vi "UHR-Fleezers Control (host) - 12.0_test_fpga_connection.vi"() -> ()   [LabVIEW 2014] (continued)
  out "Left Y":i8(slide) scale=-128.0..127.0
  out "Left X":i8(slide) scale=-128.0..127.0
  out "Right Y":i8(slide) scale=-128.0..127.0
  out "Right X":i8(slide) scale=-128.0..127.0
  out "X":bool
  out "Y":bool
  out "A":bool
  out "B":bool
  out "RB":bool
  out "LB":bool
  out "R":bool
  out "L":bool
  out "D":bool
  out "U":bool
  out "Left stick button":bool
  out "FAST Z":bool
  out "FAST X-Y":bool
  in  "XY Wait time":string="125"
  in  "Z Wait time":string="120"
  # "After"
  # "During"
  # "Trap On?"
  # "BD Flow ON?"
  # "Samp Flow ON?"
  # "Fish after\nbreak?"
  # "Thresholds (nm)"
  # "From FX (nm)"
  # "Break?"
  # "Multiple"
  # "Bad fit"
  # "Hysteresis"
  # "Trap Trig. Fl.?"
  # "1"
  # "2"
  # "Fl. Down"
  # "Fl. Up"
  # "Bead sep"
  # "Trap Display:"
  # "APD Display:"
  # "Trap Manipulation"
  # "Data Saving"
  # "DAQ"
  # "Bead Calibration"
  # "Tether screen"
  # "Bottom Pump (#1)"
  # "Central Sample Channels"
  # "Top Pump (#3)"
  # "Rate param is ul/h\nVolume param is ul"
  # "Chemyx Pump 2"
  # "Units: \n1 = ml/m\n2 = ml/h\n3 = ul/m\n4 = ul/h"
  # "X"
  # "Y"
  # "Oscillate Set 1 freq. (debugging)"
  # "BD 1"
  # "BD 2"
  # "AOD Raster Scan"
  # "Approx. trap separations"
  # "X"
  # "Y"
  # "FPGA\nreading"
  # "DMA\ntransfer"
  # "APD Gates"
  # "APD 2"
  # "APD 1"
  # "X"
  # "2D"
  # "Y"
  # "1D"
  # "Digital Out Control"
  # "Analog Out Control (Feedback Loop)"
  # "Laser Intensity Analog Input"
  # "Total AI Rates (NOT rates/trap)"
  # "(Samples/trap x Trap Sets)"
  # "(Samples/channel x\n8 if averaging (8 channels)\n4 if no averaging)"
  # "Trap 1"
  # "Trap 2"
  # "Flour./Trap 3"
  # "External Video Window"
  # "MCL Position Debugging"
  # "Temporary Control Storage\n(these used to be somewhere else, still want to keep them)"
  # "Y"
  # "X"
  # "Trap Position Difference Limits"
  # "Trap 2 (ON/OFF)"
  # "Trap 1 (ON/OFF)"
  # "Overflow happens when >40 commands\nsent in 5 sec. The 4 consecutive beeps."
  # "Try adjusting wait time to reduce 'following error threshold exceeded' occurances.\nStart by using 10ms increments."
  # "Toggles FAST Z"
  # "Toggles FAST X-Y"
  # "The default Newport max velocity is 0.4"
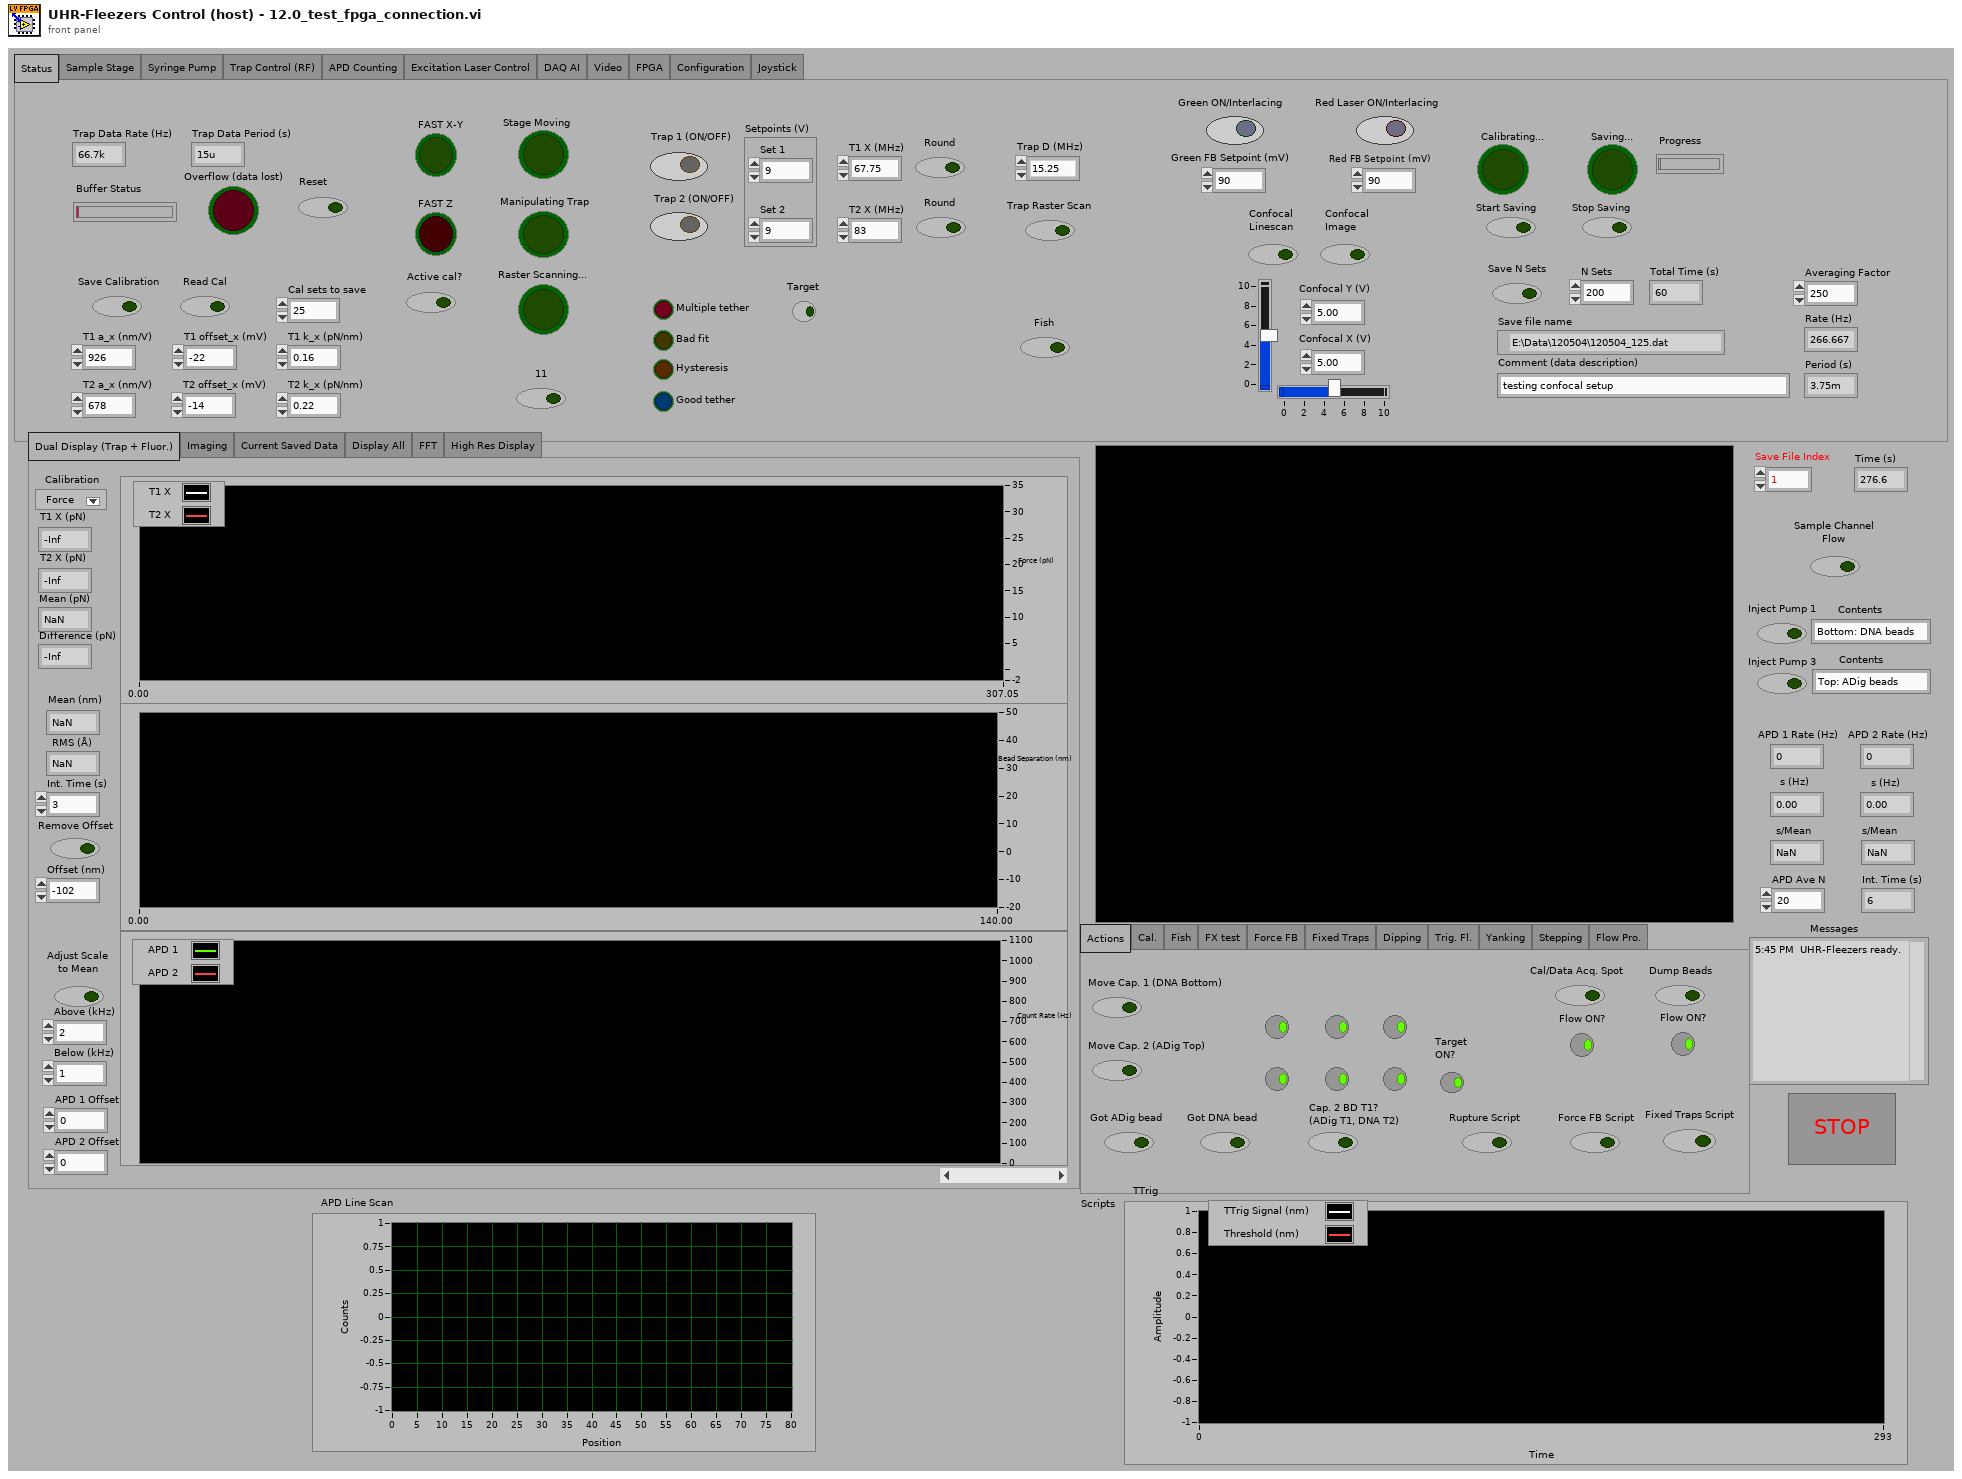
[diagram p1: front panel]
types:
  T1 = enum32{"Actions", "Cal.", "Fish", "FX test", "Force FB", "Fixed Traps", "Dipping", "Trig. Fl.", "Yanking", "Stepping", "Flow Pro."}
  T2 = typedef "IMAQ Image.ctl" = refnum<image>
  T3 = enum32{"Dual Display (Trap + Fluor.)", "Imaging", "Current Saved Data", "Display All", "FFT", "High Res Display"}
  T4 = enum32{"Status", "Sample Stage", "Syringe Pump", "Trap Control (RF)", "APD Counting", "Excitation Laser Control", "DAQ AI", "Video", "FPGA", "Configuration", "Joystick"}
  T5 = cluster{"Pump 1":cluster{"Diameter (mm)":dbl, "Units":dbl, "Volume":dbl, "Rate":dbl}, "Pump 2":cluster{"Diameter (mm)":dbl, "Units":dbl, "Volume":dbl, "Rate":dbl}, "Pump 3":cluster{"Diameter (mm)":dbl, "Units":dbl, "Volume":dbl, "Rate":dbl}}
  T6 = enum32{"IR Laser Interlacing (Direct RF Board Control Method)", "AOD Raster Scan", "Feedback on Trap Intensity", "Feedback on Trap Position"}
  T7 = typedef "LVPoint32TypeDef.ctl" = cluster{"Horizontal":i32, "Vertical":i32}
  T8 = cluster{"Scan Range AOD (nm) 2":dbl, "Step Size AOD (nm) 2":dbl, "Scan Speed AOD (nm/s) 2":dbl, "Number of scans (AOD) 2":u16, "Label":string}[]
  T9 = cluster{"Set 1":cluster{"proportional gain (Kc)":i16, "integral gain (Kc*Ts/Ti)":i16, "derivative gain (Kc*Td/Ts)":i16}, "Set 2":cluster{"proportional gain (Kc)":i16, "integral gain (Kc*Ts/Ti)":i16, "derivative gain (Kc*Td/Ts)":i16}}
  T10 = cluster{"Trap 1":fxp<+/-,16,1>, "Trap 2":fxp<+/-,16,1>}
  T11 = cluster{"proportional gain (Kc)":fxp<+/-,16,8>, "integral gain (Kc*Ts/Ti)":fxp<+/-,16,8>, "derivative gain (Kc*Td/Ts)":fxp<+/-,16,8>}
  T12 = cluster{"output high":fxp<+/-,64,32>, "output low":fxp<+/-,64,32>}
  T13 = cluster{"Set 1":fxp<+/-,16,1>, "Set 2":fxp<+/-,16,1>}
  T14 = enum32{"Main Controls", "Green laser (532 nm)", "Red laser (633 nm)"}
  T15 = cluster{"proportional gain (Kc)":i16, "integral gain (Kc*Ts/Ti)":i16, "derivative gain (Kc*Td/Ts)":i16}
  T16 = cluster{"Set 1":bool, "Set 2":bool, "Set 3":bool}
  T17 = typedef "LVMinMaxIncTypeDef.ctl" = cluster{"Minimum":dbl, "Maximum":dbl, "Increment":dbl}
  T18 = cluster{"Slow X velocity input":string, "Slow Y velocity input":string, "Fast1 X velocity input":string, "Fast1 Y velocity input":string, "Fast2 X velocity input":string, "Fast2 Y velocity input":string}
  T19 = typedef "Select Event Type.ctl" = u32
  T20 = typedef "Image Type" = u32
  T21 = typedef "nirio_resource_hc.ctl" = tag
  T22 = typedef "openfpgaref.8.6.ctl" = refnum<k20>
  T23 = cluster{"New Image":T2, "New Image":T2, "New Image":T2, "New Image":T2}
  T24 = cluster{"LB":bool, "RB":bool, "BACK":bool, "Logitech":bool, "START":bool}
  T25 = cluster{"Right X":i8, "Right Y":i8, "Left X":i8, "Left Y":i8}
  T26 = typedef "XDNodeRunTimeDep.lvlib/timing_clust.ctl" = cluster{"Expected End [f-1]":u64, "Actual End [f-1]":u64, "Finished Late? [f-1]":bool, "Expected End [i-1]":u64, "Actual End [i-1]":u64, "Finished Late? [i-1]":bool, "Expected Start [i]":u64, "Actual Start [i]":u64, "Expected Start [f]":u64, "Actual Start [f]":u64, "Source Name":string, "Structure Name":string, "Period":i64, "Deadline":i64, "Offset":i64, "Start":i64, "Priority":i32, "Timeout":i32, "Mode":T27, "Wakeup Reason":T28, "Error":errorcluster, "Source Type":string, "Secondary Source Type":string, "Global End Time":u64, "Global Start Time":u64, "Frame Duration":u64, "Iteration Duration":u64, "Assigned CPU":i32, "I/O Scan Engine Mode":u32}
  T27 = typedef "XDNodeRunTimeDep.lvlib/nitl_modes.ctl" = enum32{"No Change", "Process missed periods, maintain original phase", "Discard missed periods, maintain original phase", "Process missed periods, ignore original phase", "Discard missed periods, ignore original phase"}
  T28 = typedef "XDNodeRunTimeDep.lvlib/wakeup.ctl" = enum32{"Normal", "Aborted", "Asynchronous wakeup", "Timing source error", "Timed loop error", "Timeout"}
  T29 = enum16{"big-endian, network order", "native, host order", "little-endian"}
  T30 = enum16{"open", "replace", "create", "open or create", "replace or create", "replace or create with confirmation"}
  T31 = cluster{"Scan Range AOD (nm) 2":dbl, "Step Size AOD (nm) 2":dbl, "Scan Speed AOD (nm/s) 2":dbl, "Number of scans (AOD) 2":u16, "Label":string}
  T32 = cluster{"[0]":dbl, "[1]":dbl, "[2]":dbl, "[3]":dbl, "[4]":dbl, "[5]":dbl}
  T33 = cluster{"Diameter (mm)":dbl, "Units":dbl, "Volume":dbl, "Rate":dbl}
  T34 = enum32{"Status", "Sample Stage", "Syringe Pump", "Trap Control (RF)", "APD Counting", "Excitation Laser Control", "DAQ AI", "Video", "FPGA", "Configuration"}
  T35 = enum16{"Actions", "Cal.", "Fish", "FX test", "Force FB", "Fixed Traps", "Dipping", "Trig. Fl.", "Yanking", "Stepping", "Flow Pro."}
  T36 = cluster{"Left":i32, "Top":i32, "Width":u32, "Height":u32}
  T37 = cluster{cluster{"Left":i32, "Top":i32, "Width":u32, "Height":u32}}[]
  T38 = enum32{"setting", "request", "request control", "info", "statistics", "system settings", "I/O sub system", "HRT control", "camera descriptions", "device specific data", "event sub system settings", "event sub system results", "image memory manager"}
  T39 = typedef "AviRefnum.ctl" = refnum<k1>
  T40 = typedef "imagedata.ctl" = cluster{"image type":i32, "image depth":i32, "image":u8[], "mask":u8[], "colors":u32[], "Rectangle":cluster{"left":i16, "top":i16, "right":i16, "bottom":i16}}
  T41 = enum32{"Normal Display", "Dual Display (APD)", "FFT", "High Res Display"}
  T42 = cluster{"Origin Pixel":cluster{"X":sgl, "Y":sgl}, "Angle Relative to Horizontal (deg)":sgl, "Axis Reference":u32}
  T43 = typedef "Simple Grid Descriptor" = cluster{"X Step":sgl, "Y Step":sgl, "Unit":T44}
  T44 = typedef "Image Unit" = enum32{"Undefined", "Angström", "Micrometer", "Millimeter", "Centimeter", "Meter", "Kilometer", "Microinch", "Inch", "Feet", "Nautical miles", "Standard miles", "Steps"}
  T45 = cluster{"averaging mode":u16, "weighting mode":u16, "number of averages":u32}
  T46 = cluster{"dB On (F)":bool, "unwrap phase (F)":bool, "convert to degree (F)":bool}
  T47 = cluster{string, string, string, string, string, string, string, string}
  T48 = cluster{string, string, string, string, string, string, string, string, string, string, string, string}
  T49 = cluster{string, string, string, string, string, string, string, string, string, string, string, string, string}
  T50 = cluster{string, string, string, string, string, string, string, string, string, string, string, string, string, string}
  T51 = cluster{"BD 1 Frequency 1 (MHz)":dbl, "BD 1 Frequency 2 (MHz)":dbl}
  T52 = cluster{"f0":dbl, "df":dbl, "magnitude":dbl[]}[][]
diagram:
  w11 = T19 1073684535 items=["Service Request"=1073684491, "Trigger"=3221168138, "Clear"=1073684493, "VXI Signal"=1073684512, "VXI/VME Interrupt"=3221168161, "VXI/VME Sysfail"=1073684509, "VXI/VME Sysreset"=1073684510, "GPIB CIC"=1073684498, "GPIB Talk"=1073684499, "GPIB Listen"=1073684500, "PXI Interrupt"=1073684514, "Serial Break"=1073684515, "Serial TermChar"=1073684516, "Serial CTS"=1073684521, "Serial DSR"=1073684522, "Serial DCD"=1073684524, "Serial RI"=1073684526, "Serial Character"=1073684533, "USB Interrupt"=1073684535, "All Enabled"=1073709055] ("Event Type")
  w45 = 0.0 ("Total Volume\nFlowed P1 (uL)")
  w57 = u16 20 items=["1.0"=10, "1.5"=15, "2.0"=20] ("stop bits (10: 1 bit)")
  w60 = u16 20 items=["1.0"=10, "1.5"=15, "2.0"=20] ("stop bits (10: 1 bit)")
  w114 = u16 20 items=["1.0"=10, "1.5"=15, "2.0"=20] ("stop bits (10: 1 bit)")
  w121 = T20 2 items=["Grayscale (U8)", "Grayscale (I16)", "Grayscale (SGL)", "Complex (CSG)", "RGB (U32)", "HSL (U32)", "RGB (U64)", "Grayscale (U16)"] ("Image Type")
  w179 = cluster{"output high":i16, "output low":i16} {"output high"=3000, "output low"=0} ("FB output range 1")
  w250 = 10.0 ("y")
  w249 = 32767.0 ("y")
  w265 = 6.0  # clock mult.
  w266 = 49152000.0  # TCXO frequ.
  # "Open the RAW resource"
  # "Enable USB Interrupt Event"
  # "Safety limits on RF frequencies and amplitudes (for AOM protection)"
  # "Bottom 1 Harvard"
  # "Top 3 Harvard"
  # "Center Harvard"
  # "Bottom 1 Harvard"
  # "Top 3 Harvard"
  # "Center Harvard"
  n1 = Build Array("DIO count 1 (ticks)", "DIO count 2 (ticks)", "DIO count 3 (ticks)") -> (w166:u32[])
  n2 = local read "AO1"() -> (w244:dbl)
  n3 = local read "AO2"() -> (w243:dbl)
  n4 = local read "Scan Increment (MHz)"() -> (w261:dbl)
  n5 = local read "Continuous MCL Scanning"() -> (w231:bool)
  n6 = local read "Fast Scan Dir"() -> (w230:bool)
  n7 = local read "Number of scans (MCL)"() -> (w232:u64)
  n8 = property on="AI Count (ticks)" class="DigNum (strict)"("Val(Sgnl)"="AI Count (ticks)") -> ()  [unwired: 2 in, 2 out]
  n9 = Multiply(x=w244, y=w249) -> (x*y=w246:dbl)
  n10 = Multiply(x=w243, y=w249) -> (x*y=w248:dbl)
  n11 = Divide(x=w246, y=w250) -> (x/y=w245:dbl)
  n12 = Divide(x=w248, y=w250) -> (x/y=w247:dbl)
  n13 = To Word Integer(number=w245) -> (16bit integer=w242:i16)
  n14 = To Word Integer(number=w247) -> (16bit integer=w241:i16)
  n15 = Not(x=w230) -> (.not. x?=w225:bool)
  n16 = local read "Cycles/step (MCL)"() -> (w233:u64)
  n17 = Multiply(x=w261, y=1000.0) -> (x*y=w268:dbl)
  n18 = local read "Scan steps (MCL)"() -> (w234:u64)
  n19 = local write "Trap Pos FIFO Timeout"(u16 0 ("Trap Pos FIFO Timeout")) -> ()
  n20 = local read "Desired Scan Incr (V)"() -> (w236:dbl)
  n21 = Scale By Power Of 2(n=48, x=w268) -> (x*2^n=w269:dbl)
  n22 = Multiply(x=w266, y=w265) -> (x*y=w264:dbl)
  n23 = Divide(x=w269, y=w264) -> (x/y=w263:dbl)
  n24 = local read "Setpoints (V)"() -> (w280:cluster{"Set 1":dbl, "Set 2":dbl})
  n25 = To Quad Integer(1:w263) -> (0:w260:i64)
  n26 = Divide(x=40000000.0, y="AI Count (ticks)") -> (x/y=w221:dbl)
  n27 = Multiply(x=w236, y=32767.0) -> (x*y=w238:dbl)
  n28 = local read "Number Interlace Sets"() -> (w159:u8)
  n29 = Split 1D Array(array=w166, index=w159) -> (first subarray=w168:u32[])  [unwired: 1 out]
  n30 = Add Array Elements(numeric array=w168) -> (sum=w167:u32)
  n31 = local read "# Samples/channel"() -> (w253:u32)
  n32 = local read "Number of F/B Scans (AOD)"() -> (w254:u16)
  n33 = local read "Not-Interlacing Set"() -> (w158:enum32{"Set 1", "Set 2", "Set 3"})
  n34 = To Unsigned Byte Integer(number=w158) -> (unsigned 8bit integer=w164:u8)
  n35 = Index Array(array=w166, index=w164) -> (element=w165:u32)
  n36 = local read "Feedback On/Off"() -> (w283:cluster{"Set 1":bool, "Set 2":bool})
  n37 = local read "PID Gains"() -> (w275:T9)
  n38 = local read "Scan steps (AOD)"() -> (w259:u64)
  n39 = local read "All FB On/Off"() -> (w284:bool)
  n40 = local read "Cycles/step (AOD)"() -> (w258:u64)
  n41 = local write "AI rate (Hz)"(w221) -> ()
  n42 = Divide(x=w238, y=10.0) -> (x/y=w237:dbl)
  n43 = Multiply(x=w259, y=w258) -> (x*y=w257:u64)
  n44 = Multiply(x=3276.7, y=w280) -> (x*y=w279:cluster{"Set 1":dbl, "Set 2":dbl})
  n45 = To Word Integer(number=w237) -> (16bit integer=w235:i16)
  n46 = xnode "Open FPGA VI Reference"("resource name"=T21 "RIO1") -> ("FPGA VI Reference Out"=w43:T22, "error out"=w41:errorcluster)  [unwired: 1 in]
  n47 = Multiply(x=w257, y=u64 2) -> (x*y=w255:u64)
  n48 = local read "Sets to FIFO (Traps)"() -> (w287:T16)
  n49 = Divide(x=w221, y="FPGA Ave.") -> (x/y=w222:dbl)
  n50 = To Word Integer(number=w279) -> (16bit integer=w278:cluster{"Set 1":i16, "Set 2":i16})
  n51 = Unbundle By Name(w275) -> ("Set 1"=w274:T15, "Set 2"=w273:T15)
  n52 = Multiply(x=w255, y=w254) -> (x*y=w252:u64)
  n53 = local write "Ave. Rate (Hz)"(w222) -> ()
  n54 = Divide(x=w252, y=w253) -> (x/y=w251:dbl)
  n55 = Unbundle By Name(w278) -> ("Set 1"=w277:i16, "Set 2"=w276:i16)
  n56 = local read "2D or 1D Scan"() -> (w180:bool)
  n57 = local write "Data points/scans"(w252) -> ()
  n58 = local read "Scan BD"() -> (w270:bool)
  n59 = And(x=w283, y=w284) -> (x .and. y?=w282:cluster{"Set 1":bool, "Set 2":bool})
  n60 = local write "Data points/scan (f/b)"(w255) -> ()
  n61 = Reciprocal(x=w222) -> (1/x=w223:dbl)
  n62 = local read "N Acq Sets (Traps + Fl.)"() -> (w214:i16)
  n63 = local write "N sets should be saved"(w251) -> ()
  n64 = xnode "Invoke Method"("FPGA VI Reference In"=w43, "error in"=w41) -> ("FPGA VI Reference Out"=w178:T22, "error out"=w188:errorcluster)
  n65 = Unbundle By Name(w282) -> ("Set 1"=w286:bool, "Set 2"=w285:bool)
  n66 = local read "Interlace"() -> (w160:bool)
  n67 = Select(t=w167, s=w160, f=w165) -> (s? t:f=w157:u32)
  n68 = local write "Update Count (MCL)"(w157) -> ()
  n69 = local write "Total Counts (ticks)"(w157) -> ()
  n70 = local write "Ave. Period (s)"(w223) -> ()
  n71 = property on="2D or 1D Scan" class="Bool (strict)"("Val(Sgnl)"=w180) -> ()  [unwired: 2 in, 2 out]
  n72 = local read "APD Gate OFF Count"() -> (w84:u16)
  n73 = local read "Interlace OFF count"() -> (w87:u16)
  n74 = local read "Interlace ON count"() -> (w22:u16)
  n75 = local read "APD Gate ON Count"() -> (w80:u16)
  n76 = xnode "Read/Write Control"("FPGA VI Reference In"=w177, "error in"=w188, "ai count"="AI Count (ticks)", "Interlace ON/OFF"=w160, "Number Interlace Cycles"=w159, "AI1 Sets to FIFO"=w287, "FB On/Off Set 1"=w286, "FB On/Off Set 2"=w285, "Interlace Off Parameters"=w158, "FB Setpoint Set 1"=w277, "FB Setpoint Set 2"=w276, "FB Gains Set 1"=w274, "FB Gains Set 2"=w273, "FB output range 1"=w179, "FB output range 2"=w179, "Cycles per step"=w258, "Scan BD"=w270, "Number of scans"=w254, "Scan steps"=w259, "Scan freq.  increment"=w260, "AO1"=w242, "AO2"=w241, "Scan freq.  increment (MCL)"=w235, "Scan steps (MCL)"=w234, "Cycles per step (MCL)"=w233, "Number of scans (MCL)"=w232, "MCL count"=w157, "Cont. Scan (MCL)"=w231, "MCL Scan Axis"=w225, "1D or 2D Scan?"=w180, "N of AI1 Int Acq Sets"=w214, "Freq or Amp switch first"="Freq or Amp switch first", "Freq switch delay"="Freq switch delay", "Amp switch delay"="Amp switch delay", "Swap F1 and F2"="Swap F1 and F2", "APD to FIFO"=FALSE, "DIO count 1 (ticks)"="DIO count 1 (ticks)", "DIO count 2 (ticks)"="DIO count 2 (ticks)", "DIO count 3 (ticks)"="DIO count 3 (ticks)") -> ("FPGA VI Reference Out"=w91:T22, "error out"=w89:errorcluster)  [unwired: 1 in]
  n77 = local read "Duty frequency (ON 1/N cycles)"() -> (w86:u16)
  n78 = local read "APD Integration Time (s)"() -> (w72:dbl)
  n79 = local read "DMA Update Period (s)"() -> (w71:dbl)
  n80 = local read "Red Laser ON/Interlacing"() -> (w25:bool)
  n81 = Add(x=w80, y=w84) -> (x+y=w82:u16)
  n82 = local read "Laser interlacing mode (all lasers)"() -> (w24:enum32{"Laser ON", "Laser OFF", "Interlace"})
  n83 = Add(x=w22, y=w87) -> (x+y=w85:u16)
  n84 = local read "Green ON/Interlacing"() -> (w156:bool)
  n85 = Multiply(x=w82, y=w86) -> (x*y=w83:u16)
  n86 = Multiply(x="Red FB Setpoint (mV)", y=3.2767) -> (x*y=w15:dbl)
  n87 = Multiply(x=w86, y=w85) -> (x*y=w79:u16)
  n88 = Reciprocal(x=w72) -> (1/x=w69:dbl)
  n89 = Multiply(x=w72, y=40000000.0) -> (x*y=w68:dbl)
  n90 = Divide(x=w71, y=w72) -> (x/y=w74:dbl)
  n91 = Multiply(x="Green intensity % (FB OFF)", y=655.35) -> (x*y=w146:dbl)
  n92 = local read "Invert laser interlacing"() -> (w20:bool)
  n93 = case shown="False" w25 {
    tunnel: w24 -> [_ w311]
    tunnel: [enum32{"Laser ON", "Laser OFF", "Interlace"}."Laser OFF" ("Laser interlacing mode (all lasers)") w311] -> w23
    frame False {
    }
    frame True {
    }
  }
  n94 = local read "Invert APD Gate"() -> (w78:bool)
  n95 = Multiply(x="Green FB Setpoint (mV)", y=3.2767) -> (x*y=w143:dbl)
  n96 = local read "APD Gate"() -> (w77:enum32{"ON", "OFF", "Interlace"})
  n97 = Subtract(x=w83, y=w80) -> (x-y=w81:u16)
  n98 = To Word Integer(number=w15) -> (16bit integer=w14:i16)
  n99 = local write "Green FB Count"(w79) -> ()
  n100 = local write "APD Acq Rate (Hz)"(w69) -> ()
  n101 = To Unsigned Long Integer(number=w68) -> (unsigned 32bit integer=w66:u32)
  n102 = Multiply(x=2.0, y=w74) -> (x*y=w73:dbl)
  n103 = To Unsigned Word Integer(number=w146) -> (unsigned 16bit integer=w144:u16)
  n104 = Subtract(x=w79, y=w22) -> (x-y=w21:u16)
  n105 = local write "APD Samples/FIFO Acq."(w74) -> ()
  n106 = To Word Integer(number=w143) -> (16bit integer=w141:i16)
  n107 = local write "APD Elements/DMA read"(w73) -> ()
  n108 = case shown="False" w156 {
    tunnel: w24 -> [_ w313]
    tunnel: [enum32{"Laser ON", "Laser OFF", "Interlace"}."Laser OFF" ("Green laser mode") w313] -> w26
    frame False {
    }
    frame True {
    }
  }
  n109 = local write "APD Int. Count"(w66) -> ()
  n110 = Multiply(x="Red intensity % (FB OFF)", y=655.35) -> (x*y=w30:dbl)
  n111 = local read "Trap Pos. AI1 X Pre-scale"() -> (w101:u16)
  n112 = local read "Trap Pos FB Monitor\nT1 or T2"() -> (w108:bool)
  n113 = To Unsigned Word Integer(number=w30) -> (unsigned 16bit integer=w29:u16)
  n114 = local read "Trap Pos FB Int Count"() -> (w95:u16)
  n115 = local read "APD 1 AO Mult."() -> (w76:i16)
  n116 = local read "Trap Pos FB Negate Action"() -> (w107:bool)
  n117 = local read "APD 2 AO Mult."() -> (w75:i16)
  n118 = local read "Trap Pos. FB Offset Factor"() -> (w106:i64)
  n119 = local read "Trap Pos. FB Mult Factor"() -> (w105:i64)
  n120 = local read "Differential FB?"() -> (w63:bool)
  n121 = local read "Neg. TTrig FPGA"() -> (w65:bool)
  n122 = local read "Trap Pos. FB Gains"() -> (w103:T11)
  n123 = local read "Trap Pos. FB Range"() -> (w104:T12)
  n124 = xnode "Read/Write Control"("FPGA VI Reference In"=w91, "error in"=w89, "Invert APD Gate"=w78, "APD Gate ON Count"=w80, "APD Gate OFF Count"=w81, "APD Acq Rate Count"=w66, "APD Gate Operating Mode"=w77, "APD 1 AO scale factor"=w76, "APD 2 AO scale factor"=w75, "Green interlace ON count"=w22, "Green interlace OFF count"=w21, "Green interlace ON count 2"=w22, "Green interlace OFF count 2"=w21, "Green FB Count"=w79, "RI ON count"=w22, "RI OFF count"=w21) -> ("FPGA VI Reference Out"=w90:T22, "error out"=w88:errorcluster)
  n125 = xnode "Read/Write Control"("FPGA VI Reference In"=w90, "error in"=w88, "Invert GI 2"=w20, "Operating Mode 2"=w26, "Green FB Gains"="Green FB Gains", "Green FB Setpoint"=w141, "Green FB On/Off"="Green FB On/Off", "Current Out"=w144, "Green int current ON count adj"="Green int current ON count adj", "Operating Mode"=w26, "Invert GI"=w20, "Trap Pos FB Monitor T1 or T2"=w108, "Trap Pos FB Negate Action"=w107, "Trap Pos. FB Offset Factor"=w106, "Trap Pos. FB Mult Factor"=w105, "Trap Pos. FB Range"=w104, "Trap Pos. FB Gains"=w103, "Force feedback"=FALSE, "AI1 X Scale"=w101, "Trap Pos to FIFO"=TRUE, "Trap Pos FB Int Count"=w95, "TTrig Negate Pos"=w65, "FB Trig Integrate"="FB Trig Integrate", "Diff FB Measurement?"=w63, "Negate Diff?"="Negate Diff?", "RI Current Out"=w29, "Red operating mode"=w23, "RI operating mode 2"=w23, "Invert RI"=w20, "Invert RI 2"=w20, "Red FB Gains"="Red FB Gains", "Red FB On/Off"="Red FB On/Off", "Red FB Setpoint"=w14) -> ("FPGA VI Reference Out"=w154:T22, "error out"=w155:errorcluster)
  n126 = xnode "Invoke Method"("FPGA VI Reference In"=w154, "error in"=w155, "Requested Depth"="Trap AI FIFO Depth") -> ("FPGA VI Reference Out"=w110:T22, "error out"=w109:errorcluster)  [unwired: 1 out]
  n127 = xnode "Invoke Method"("FPGA VI Reference In"=w110, "error in"=w109, "Requested Depth"="Trap Position FIFO Depth") -> ("FPGA VI Reference Out"=w97:T22, "error out"=w96:errorcluster)  [unwired: 1 out]
  n128 = flat-sequence {
    tunnel: w178 -> [w318]
    tunnel: [w318] -> w177
    tunnel: [w317] -> w176
    tunnel: [w316] -> w175
    tunnel: [w314] -> w173
    tunnel: [w315] -> w174
    frame #0 {
      w315 = T17 {"Minimum"=0.0, "Maximum"=40.0, "Increment"=1.0} ("Min Max Inc")
      w314 = T17 {"Minimum"=0.0, "Maximum"=50.0, "Increment"=1.0} ("Data Entry Limits")
      w317 = T17 {"Minimum"=60.0, "Maximum"=90.0, "Increment"=1.0} ("Min Max Inc")
      w316 = T17 {"Minimum"=0.0, "Maximum"=50.0, "Increment"=1.0} ("Data Entry Limits")
      n129 = property on="BD 2 Frequency 1 (MHz)" class="DigNum (strict)"("Data Range"=w315) -> ()  [unwired: 2 in, 2 out]
      n130 = property on="BD 2 Frequency 3 (MHz)" class="DigNum (strict)"("Data Range"=w315) -> ()  [unwired: 2 in, 2 out]
      n131 = property on="BD 2 Frequency 2 (MHz)" class="DigNum (strict)"("Data Range"=w315) -> ()  [unwired: 2 in, 2 out]
      n132 = property on="BD 1 Frequency 1 (MHz)" class="DigNum (strict)"("Data Range"=w317) -> ()  [unwired: 2 in, 2 out]
      n133 = property on="BD 1 Frequency 2 (MHz)" class="DigNum (strict)"("Data Range"=w317) -> ()  [unwired: 2 in, 2 out]
      n134 = property on="BD 1 Frequency 3 (MHz)" class="DigNum (strict)"("Data Range"=w317) -> ()  [unwired: 2 in, 2 out]
      n135 = property on="BD 2 Amplitude 1 (%)" class="DigNum (strict)"("Data Range"=w314) -> ()  [unwired: 2 in, 2 out]
      n136 = property on="BD 2 Amplitude 2 (%)" class="DigNum (strict)"("Data Range"=w314) -> ()  [unwired: 2 in, 2 out]
      n137 = property on="BD 2 Amplitude 3 (%)" class="DigNum (strict)"("Data Range"=w314) -> ()  [unwired: 2 in, 2 out]
      n138 = property on="BD 1 Amplitude 3 (%)" class="DigNum (strict)"("Data Range"=w316) -> ()  [unwired: 2 in, 2 out]
      n139 = property on="BD 1 Amplitude 2 (%)" class="DigNum (strict)"("Data Range"=w316) -> ()  [unwired: 2 in, 2 out]
      n140 = property on="BD 1 Amplitude 1 (%)" class="DigNum (strict)"("Data Range"=w316) -> ()  [unwired: 2 in, 2 out]
      "X RF Frequency Limits (MHz)" <- w317
      "X RF Amplitude Limits (%)" <- w316
      "Y RF Amplitude Limits (%)" <- w314
      "Y RF Frequency Limits (MHz)" <- w315
    }
  }
  n141 = xnode "Invoke Method"("FPGA VI Reference In"=w97, "error in"=w96) -> ("FPGA VI Reference Out"=w187:T22, "error out"=w186:errorcluster)  [unwired: 1 in]
  n142 = flat-sequence "Initial FPGA Loop Relative Phase Adjustment" {
    tunnel: "Initial Phase Adjustment (APD 2 Gate)" -> [w321]
    tunnel: "Initial Phase Adjust (GI) 2" -> [w322]
    tunnel: "Initial Phase Adj. (MCL)" -> [w320]
    tunnel: w186 -> [w323]
    tunnel: w187 -> [w324]
    tunnel: "Initial Phase Adjust (GI)" -> [w325]
    tunnel: "Initial Phase Adjustment (AI1)" -> [w326]
    tunnel: [w326] -> w40
    tunnel: [w325] -> w39
    tunnel: [w324] -> w38
    tunnel: [w323] -> w37
    tunnel: [w320] -> w36
    tunnel: [w322] -> w35
    tunnel: [w321] -> w34
    tunnel: [w339] -> w196
    tunnel: [w333] -> w192
    tunnel: "Initial Phase Adjustment (APD Acq)" -> [w332]
    tunnel: "Initial Phase Adjustment (APD 1 Gate)" -> [w331]
    tunnel: "Initial Phase Adjust (Green FB)" -> [w330]
    tunnel: w40 -> [w338]
    tunnel: w39 -> [w337]
    tunnel: w38 -> [w336]
    tunnel: w37 -> [w335]
    tunnel: w36 -> [w334]
    tunnel: w35 -> [w329]
    tunnel: w34 -> [w328]
    tunnel: "Initial Phase Adjustment (RI)" -> [w327]
    tunnel: w196 -> [w341]
    tunnel: [w342] -> w193
    tunnel: w192 -> [w342]
    tunnel: [w341] -> w191
    tunnel: w193 -> [w345]
    tunnel: w191 -> [w344]
    tunnel: [w347] -> w190
    tunnel: [w346] -> w189
    tunnel: [w349] -> w194
    tunnel: [w350] -> w195
    tunnel: w190 -> [w350]
    tunnel: w189 -> [w349]
    frame #0 {
      n143 = Wait (ms)(milliseconds to wait=u32 100) -> ()  [unwired: 1 out]
    }
    frame #1 {
      n144 = xnode "Read/Write Control"("FPGA VI Reference In"=w336, "error in"=w335, "Phase count adjustment"=w338, "Phase count adjustment (GI)"=w337, "Phase count adjustment (MCL)"=w334, "Phase Count Adjustment (APD Acq)"=w332, "Phase count adjustment (APD 1 Gate)"=w331, "Phase count adjustment (APD 2 Gate)"=w328, "Phase count adjustment (Green FB)"=w330, "Phase count adjustment (GI) 2"=w329, "Phase count adjustment (RI)"=w327) -> ("FPGA VI Reference Out"=w333:T22, "error out"=w339:errorcluster)
    }
    frame #2 {
      n145 = Wait (ms)(milliseconds to wait=u32 100) -> ()  [unwired: 1 out]
    }
    frame #3 {
      w343 = TRUE
      n146 = xnode "Read/Write Control"("FPGA VI Reference In"=w345, "error in"=w344, "+ phase"=w343, "+ phase (GI)"=w343, "+ phase (MCL)"=w343, "+ phase (APD Acq)"=w343, "+ phase (APD 1 Gate)"=w343, "+ phase (APD 2 Gate)"=w343, "+ phase (Green FB)"=w343, "+ phase (GI) 2"=w343, "+ phase (RI)"=w343) -> ("FPGA VI Reference Out"=w346:T22, "error out"=w347:errorcluster)
    }
    frame #4 {
      n147 = Wait (ms)(milliseconds to wait=u32 100) -> ()  [unwired: 1 out]
    }
  }
  n148 = VISA Open(VISA resource name=refnum<visa-resource-name> "USB0::0x046D::0xC21D::F3DA24A3::RAW" ("USB port")) -> (VISA resource name=w13:refnum<visa-resource-name>, error out=w12:errorcluster)  [unwired: 1 in, 3 out]
  n149 = local read "Phase adj. (Green FB)"() -> (w169:i16)
  n150 = local read "Phase adj. (GI) 2"() -> (w147:i16)
  n151 = local read "Phase adj. (RI)"() -> (w27:i16)
  n152 = local read "Phase adjust (MCL)"() -> (w226:i16)
  n153 = local read "Phase adj. (AI1)"() -> (w228:i16)
  n154 = local read "Phase adj. (GI)"() -> (w227:i16)
  n155 = VISA Enable Event(8:w12, 10:w11, 11:w13) -> (0:w8:errorcluster, 3:w7:refnum<visa-resource-name>)  [unwired: 1 out]
  n156 = xnode "Read/Write Control"("FPGA VI Reference In"=w194, "error in"=w195, "Phase count adjustment"=w228, "Phase count adjustment (GI)"=w227, "Phase count adjustment (MCL)"=w226, "Phase Count Adjustment (APD Acq)"="Phase Adj. (APD Acq)", "Phase count adjustment (APD 1 Gate)"="Phase Adj. (APD 1 Gate)", "Phase count adjustment (APD 2 Gate)"="Phase Adj. (APD 2 Gate)", "Phase count adjustment (Green FB)"=w169, "Phase count adjustment (GI) 2"=w147, "Phase count adjustment (RI)"=w27) -> ("FPGA VI Reference Out"=w42:T22, "error out"=w203:errorcluster)
  n157 = call "Initialize RF boards - interlace 3.vi"("error in"=w203, "FPGA VI Reference In"=w42) -> ("error out"=w201:errorcluster, "FPGA VI Reference Out"=w202:T22)
  n158 = call "set RF board frequency - interlace.vi"("Board 2 Frequency Limits"=w174, "Board 1 Frequency Limits"=w176, "error in"=w201, "FPGA VI Reference In"=w202, "Board 2 Frequency 3 (MHz)"="BD 2 Frequency 3 (MHz)", "Board 1 Frequency 3 (MHz)"="BD 1 Frequency 3 (MHz)", "Board 2 Frequency 2 (MHz)"="BD 2 Frequency 2 (MHz)", "Board 2 Frequency 1 (MHz)"="BD 2 Frequency 1 (MHz)", "Board 1 Frequency 2 (MHz)"="BD 1 Frequency 2 (MHz)", "Board 1 Frequency 1  (MHz)"="BD 1 Frequency 1 (MHz)") -> ("error out"=w302:errorcluster, "FPGA VI Reference Out"=w303:T22)
  n159 = call "set RF board amplitude - interlace.vi"("Board 2 Amplitude Limits"=w173, "Board 1 Amplitude Limits"=w175, "error in"=w302, "FPGA VI Reference In"=w303, "Board 2 Amplitude 3 (%)"="BD 2 Amplitude 3 (%)", "Board 1 Amplitude 3 (%)"="BD 1 Amplitude 3 (%)", "Board 2 Amplitude 2 (%)"="BD 2 Amplitude 2 (%)", "Board 2 Amplitude 1 (%)"="BD 2 Amplitude 1 (%)", "Board 1 Amplitude 2 (%)"="BD 1 Amplitude 2 (%)", "Board 1 Amplitude 1 (%)"="BD 1 Amplitude 1 (%)") -> ("error out"=w290:errorcluster, "FPGA VI Reference Out"=w291:T22)
  n160 = flat-sequence {
    tunnel: w291 -> [w360]
    tunnel: w290 -> [w359]
    tunnel: [w358] -> w295
    tunnel: [w357] -> w294
    tunnel: [w364] -> w293
    tunnel: w295 -> [w364]
    tunnel: [w363] -> w292
    tunnel: w294 -> [w363]
    tunnel: w293 -> [w373]
    tunnel: w292 -> [w372]
    tunnel: [w371] -> w51
    tunnel: [w370] -> w98
    frame #0 {
      w351 = FALSE ("Retract Pump 3")
      n161 = local read "Trap 1 (ON/OFF)"() -> (w352:bool)
      n162 = xnode "Read/Write Control"("FPGA VI Reference In"=w360, "error in"=w359, "Direct RF Box  Communication"=FALSE) -> ("FPGA VI Reference Out"=w358:T22, "error out"=w357:errorcluster)
      n163 = local write "Saving..."(FALSE ("Saving Data")) -> ()
      n164 = local write "Stop All"(FALSE ("Stop All")) -> ()
      n165 = local write "Retract Pump 1"(w351) -> ()
      n166 = local write "Retract Pump 3"(w351) -> ()
      n167 = local write "Index"(1.0 ("Index")) -> ()
      n168 = property on="Trap 1 ON" class="Bool (strict)"("Value"=w352) -> ()  [unwired: 2 in, 2 out]
      "Manipulating Trap" <- FALSE ("Manipulating Trap")
    }
    frame #1 {
      n169 = local read "Trap 2 (ON/OFF)"() -> (w362:bool)
      n170 = Wait (ms)(milliseconds to wait=u32 10) -> ()  [unwired: 1 out]
      n171 = property on="Trap 2 ON" class="Bool (strict)"("Val(Sgnl)"=w362) -> ()  [unwired: 2 in, 2 out]
    }
    frame #2 {
      n172 = local read "Scan Range (nm)"() -> (w366:dbl)
      n173 = xnode "Read/Write Control"("FPGA VI Reference In"=w373, "error in"=w372, "FPGA Controls  RF Box"=TRUE ("Direct RF Box  Communication")) -> ("FPGA VI Reference Out"=w371:T22, "error out"=w370:errorcluster)
      n174 = call "Update messages.vi"("Message to add"="UHR-Fleezers ready.", "Old message string"="") -> ("New message string"=w369:string)
      n175 = local write "Messages"(w369) -> ()
      n176 = property on="Scan Range (nm)" class="DigNum (strict)"("Val(Sgnl)"=w366) -> ()  [unwired: 2 in, 2 out]
    }
  }
  n177 = Subtract(x="BD 1 Frequency 1 (MHz)", y="BD 1 Frequency 2 (MHz)") -> (x-y=w213:dbl)
  n178 = Subtract(x="BD 2 Frequency 1 (MHz)", y="BD 2 Frequency 2 (MHz)") -> (x-y=w212:dbl)
  n179 = Square(x=w212) -> (x^2=w210:dbl)
  n180 = Square(x=w213) -> (x^2=w211:dbl)
  n181 = Add(x=w211, y=w210) -> (x+y=w209:dbl)
  n182 = Square Root(x=w209) -> (sqrt(x)=w208:dbl)
  n183 = local write "Trap D (MHz)"(w208) -> ()
  n184 = call "IMAQ Create"("Image Name"="APD 1 Image", "Image Type"=w121) -> ("New Image"=w120:T2)  [unwired: 3 in, 1 out]
  n185 = call "IMAQ Create"("Image Name"="APD 2 Image", "Image Type"=w121) -> ("New Image"=w119:T2)  [unwired: 3 in, 1 out]
  n186 = call "IMAQ Create"("Image Name"="Det. X Image", "Image Type"=w121) -> ("New Image"=w118:T2)  [unwired: 3 in, 1 out]
  n187 = call "IMAQ Create"("Image Name"="Det. Y Image", "Image Type"=w121) -> ("New Image"=w117:T2)  [unwired: 3 in, 1 out]
  n188 = Bundle("New Image"=w120, "New Image"=w119, "New Image"=w118, "New Image"=w117) -> (w116:T23)  [unwired: 1 in]
  n189 = call-poly "VISA Configure Serial Port"("VISA resource name"="Bottom  1 Harvard Syringe Pump Serial Port", "baud rate (9600)"=u32 115200, "stop bits (10: 1 bit)"=w57) -> ("VISA resource name out"=w53:refnum<visa-resource-name>, "error out"=w52:errorcluster)  [unwired: 4 in, 7 out]
  n190 = call-poly "VISA Configure Serial Port"("VISA resource name"="Top 3 Harvard Syringe Pump Serial Port", "baud rate (9600)"=u32 115200, "stop bits (10: 1 bit)"=w60) -> ("VISA resource name out"=w55:refnum<visa-resource-name>, "error out"=w54:errorcluster)  [unwired: 4 in, 7 out]
  n191 = call-poly "VISA Configure Serial Port"("VISA resource name"="Sample Chamber Stage Serial Port", "baud rate (9600)"=u32 19200) -> ("VISA resource name out"=w5:refnum<visa-resource-name>, "error out"=w130:errorcluster)  [unwired: 4 in, 8 out]
  "Stage Control Serial Error" <- w130
  n192 = while {
    shift-right: [w393] -> w4
    shift-left: w8 -> [w394]
    shift-right: [w391] -> w3
    shift-left: w7 -> [w392]
    tunnel: w5 -> [w390]
    stop <- w395 stop-if-true
    n193 = global read "FAST_Global_var.vi" "FAST L"() -> (→"FAST Z" →"FAST Z":bool)
    n194 = global read "FAST_Global_var.vi" "FAST R"() -> (→"FAST X-Y" →"FAST X-Y":bool)
    n195 = call "LogitechSubVi.vi"("USB port"=w392, "VISA resource name in 2 (for the Newport)"=w390, "error in (no error)"=w394, "X-Y Wait time"="XY Wait time", "Z Wait time"="Z Wait time", "XY Speed Definitions"="XY Speed Definitions", "Z Speed Definitions"="Z Speed Definitions") -> ("Right stick button"=→"Right stick button":bool, "Left stick button"=→"Left stick button":bool, "USB port out"=w391:refnum<visa-resource-name>, "error out"=w393:errorcluster, "A B X Y"=w378:cluster{"A":bool, "B":bool, "X":bool, "Y":bool}, "LB RB"=w389:T24, "U D L R"=w379:cluster{"U":bool, "D":bool, "L":bool, "R":bool}, "Sticks"=w386:T25)  [unwired: 5 in]
    n196 = Unbundle By Name(w379) -> ("U"=→"U":bool, "D"=→"D":bool, "L"=→"L":bool, "R"=→"R":bool)
    n197 = Unbundle By Name(w389) -> ("LB"=w377:bool, "RB"=w376:bool, "BACK"=→"BACK":bool, "Logitech"=w375:bool, "START"=→"START":bool)
    "LB" <- w376
    "RB" <- w377
    "Logitech" <- w375
    n198 = case shown="True" w376 {
      frame False {
      }
      frame True {
        n199 = local read "Trap 1 (ON/OFF)"() -> (w420:bool)
        n200 = Not(x=w420) -> (.not. x?=w421:bool)
        n201 = property on="Trap 1 (ON/OFF)" class="Bool (strict)"("Val(Sgnl)"=w421) -> ()  [unwired: 2 in, 2 out]
      }
    }
    n202 = local write "Save Image"(w375) -> ()
    n203 = case shown="True" w377 {
      frame False {
      }
      frame True {
        n204 = local read "Trap 2 (ON/OFF)"() -> (w418:bool)
        n205 = Not(x=w418) -> (.not. x?=w419:bool)
        n206 = property on="Trap 2 (ON/OFF)" class="Bool (strict)"("Val(Sgnl)"=w419) -> ()  [unwired: 2 in, 2 out]
      }
    }
    n207 = Unbundle By Name(w386) -> ("Right X"=w415:i8, "Right Y"=w414:i8, "Left X"=w412:i8, "Left Y"=w410:i8)
    n208 = Not Equal To 0?(x=w415) -> (x != 0?=w417:bool)
    n209 = Not Equal To 0?(x=w410) -> (x != 0?=w411:bool)
    n210 = Not Equal To 0?(x=w412) -> (x != 0?=w413:bool)
    n211 = Unbundle By Name(w378) -> ("A"=w402:bool, "B"=w400:bool, "X"=w398:bool, "Y"=w396:bool)
    "B" <- w400
    "A" <- w402
    "Y" <- w396
    "X" <- w398
    n212 = case shown="\"Got ADig\", Default" "A command" {
      tunnel: w402 -> [w449 w451 w453 w456]
      frame "Got ADig", Default {
        n213 = case shown="True" w449 {
          selector: w449 -> [_ w450]
          frame False {
          }
          frame True {
            n214 = property on="Got ADig bead" class="Bool (strict)"("Val(Sgnl)"=w450) -> ()  [unwired: 2 in, 2 out]
          }
        }
      }
      frame "Dump" {
        n215 = case shown="True" w451 {
          selector: w451 -> [_ w452]
          frame False {
          }
          frame True {
            n216 = property on="Dump Beads" class="Bool (strict)"("Val(Sgnl)"=w452) -> ()  [unwired: 2 in, 2 out]
          }
        }
      }
      frame "Fish" {
        n217 = case shown="True" w453 {
          frame False {
          }
          frame True {
            n218 = local read "Fish"() -> (w454:bool)
            n219 = Not(x=w454) -> (.not. x?=w455:bool)
            n220 = property on="Fish" class="Bool (strict)"("Val(Sgnl)"=w455) -> ()  [unwired: 2 in, 2 out]
          }
        }
      }
      frame "Got DNA" {
        n221 = case shown="True" w456 {
          selector: w456 -> [_ w457]
          frame False {
          }
          frame True {
            n222 = property on="Got DNA bead" class="Bool (strict)"("Val(Sgnl)"=w457) -> ()  [unwired: 2 in, 2 out]
          }
        }
      }
    }
    n223 = case shown="\"Got DNA\", Default" "B command" {
      tunnel: w400 -> [w440 w442 w444 w446]
      frame "Got DNA", Default {
        n224 = case shown="True" w440 {
          selector: w440 -> [_ w441]
          frame False {
          }
          frame True {
            n225 = property on="Got DNA bead" class="Bool (strict)"("Val(Sgnl)"=w441) -> ()  [unwired: 2 in, 2 out]
          }
        }
      }
      frame "Got ADig" {
        n226 = case shown="True" w442 {
          selector: w442 -> [_ w443]
          frame False {
          }
          frame True {
            n227 = property on="Got ADig bead" class="Bool (strict)"("Val(Sgnl)"=w443) -> ()  [unwired: 2 in, 2 out]
          }
        }
      }
      frame "Dump" {
        n228 = case shown="True" w444 {
          selector: w444 -> [_ w445]
          frame False {
          }
          frame True {
            n229 = property on="Dump Beads" class="Bool (strict)"("Val(Sgnl)"=w445) -> ()  [unwired: 2 in, 2 out]
          }
        }
      }
      frame "Fish" {
        n230 = case shown="True" w446 {
          frame False {
          }
          frame True {
            n231 = local read "Fish"() -> (w447:bool)
            n232 = Not(x=w447) -> (.not. x?=w448:bool)
            n233 = property on="Fish" class="Bool (strict)"("Val(Sgnl)"=w448) -> ()  [unwired: 2 in, 2 out]
          }
        }
      }
    }
    n234 = Not Equal To 0?(x=w414) -> (x != 0?=w416:bool)
    n235 = case shown="True" w417 {
      tunnel: w415 -> [_ w461]
      frame False {
      }
      frame True {
        "Right X" <- w461
      }
    }
    n236 = case shown="True" w411 {
      tunnel: w410 -> [_ w458]
      frame False {
      }
      frame True {
        "Left Y" <- w458
      }
    }
    n237 = case shown="True" w416 {
      tunnel: w414 -> [_ w460]
      frame False {
      }
      frame True {
        "Right Y" <- w460
      }
    }
    n238 = case shown="\"Dump\", Default" "X command" {
      tunnel: w398 -> [w431 w433 w436 w438]
      frame "Dump", Default {
        n239 = case shown="True" w431 {
          selector: w431 -> [_ w432]
          frame False {
          }
          frame True {
            n240 = property on="Dump Beads" class="Bool (strict)"("Val(Sgnl)"=w432) -> ()  [unwired: 2 in, 2 out]
          }
        }
      }
      frame "Fish" {
        n241 = case shown="True" w433 {
          frame False {
          }
          frame True {
            n242 = local read "Fish"() -> (w434:bool)
            n243 = Not(x=w434) -> (.not. x?=w435:bool)
            n244 = property on="Fish" class="Bool (strict)"("Val(Sgnl)"=w435) -> ()  [unwired: 2 in, 2 out]
          }
        }
      }
      frame "Got ADig" {
        n245 = case shown="True" w436 {
          selector: w436 -> [_ w437]
          frame False {
          }
          frame True {
            n246 = property on="Got ADig bead" class="Bool (strict)"("Val(Sgnl)"=w437) -> ()  [unwired: 2 in, 2 out]
          }
        }
      }
      frame "Got DNA" {
        n247 = case shown="True" w438 {
          selector: w438 -> [_ w439]
          frame False {
          }
          frame True {
            n248 = property on="Got DNA bead" class="Bool (strict)"("Val(Sgnl)"=w439) -> ()  [unwired: 2 in, 2 out]
          }
        }
      }
    }
    n249 = case shown="True" w413 {
      tunnel: w412 -> [_ w459]
      frame False {
      }
      frame True {
        "Left X" <- w459
      }
    }
    n250 = case shown="\"Fish\", Default" "Y command" {
      tunnel: w396 -> [w422 w425 w427 w429]
      frame "Fish", Default {
        n251 = case shown="True" w422 {
          frame False {
          }
          frame True {
            n252 = local read "Fish"() -> (w423:bool)
            n253 = Not(x=w423) -> (.not. x?=w424:bool)
            n254 = property on="Fish" class="Bool (strict)"("Val(Sgnl)"=w424) -> ()  [unwired: 2 in, 2 out]
          }
        }
      }
      frame "Dump" {
        n255 = case shown="True" w425 {
          selector: w425 -> [_ w426]
          frame False {
          }
          frame True {
            n256 = property on="Dump Beads" class="Bool (strict)"("Val(Sgnl)"=w426) -> ()  [unwired: 2 in, 2 out]
          }
        }
      }
      frame "Got ADig" {
        n257 = case shown="True" w427 {
          selector: w427 -> [_ w428]
          frame False {
          }
          frame True {
            n258 = property on="Got ADig bead" class="Bool (strict)"("Val(Sgnl)"=w428) -> ()  [unwired: 2 in, 2 out]
          }
        }
      }
      frame "Got DNA" {
        n259 = case shown="True" w429 {
          selector: w429 -> [_ w430]
          frame False {
          }
          frame True {
            n260 = property on="Got DNA bead" class="Bool (strict)"("Val(Sgnl)"=w430) -> ()  [unwired: 2 in, 2 out]
          }
        }
      }
    }
    n261 = local read "Stop All"() -> (w395:bool)
  }
  n262 = VISA Close(VISA resource name=w3, error in (no error)=w4) -> (error out=w9:errorcluster)
  n263 = call <vilib>:"Simple Error Handler.vi"("error in (no error)"=w9) -> ()  [unwired: 1 in, 8 out]
  n264 = call-poly "VISA Configure Serial Port"("VISA resource name"="Center Harvard Syringe Pump Serial Port", "baud rate (9600)"=u32 115200, "stop bits (10: 1 bit)"=w114) -> ("VISA resource name out"=w111:refnum<visa-resource-name>, "error out"=w112:errorcluster)  [unwired: 4 in, 7 out]
  n265 = disable-structure shown="Disabled" {
    disable-tunnel: [w463 _] -> w272
    disable-tunnel: w51 -> [w462 _]
    frame Disabled {
      n266 = node-c288() -> (w465:T26)  [unwired: 4 out]
      n267 = timed-loop "Rough control of MCL mirror stage (debugging)" {
        tunnel: w462 -> [w468]
        tunnel: [w467] -> w463
        timing: w465 -> [_]
        timing-out: [_] -> w464
        stop <- w467 stop-if-true
        n268 = node-c288() -> ()  [unwired: 2 out]
        n269 = case shown="1" "MCL Mode" {
          tunnel: w468 -> [_ w471 w518]
          frame 0, Default {
          }
          frame 1 {
            n270 = node-c288() -> (w473:T26)  [unwired: 4 out]
            n271 = timed-loop "Oscillate MCL mirror" {
              timing: w473 -> [_]
              timing-out: [_] -> w472
              tunnel: w471 -> [w512]
              i -> [w511]
              stop <- w474 stop-if-true
              n272 = node-c288() -> (w510:i64)  [unwired: 1 out]
              n273 = Multiply(x="AO1", y=32767.0) -> (x*y=w506:dbl)
              n274 = Multiply(x="AO2", y=32767.0) -> (x*y=w501:dbl)
              n275 = Divide(x=w506, y=10.0) -> (x/y=w507:dbl)
              n276 = Divide(x=w501, y=10.0) -> (x/y=w502:dbl)
              n277 = To Word Integer(number=w507) -> (16bit integer=w499:i16)
              n278 = To Word Integer(number=w502) -> (16bit integer=w498:i16)
              n279 = Divide(x=w510, y=i64 1000) -> (x/y=w481:dbl)
              n280 = Multiply(x=w481, y=w511) -> (x*y=w492:dbl)
              n281 = Multiply(x="Osc. freq. (Hz) 2", y=6.283185307179586) -> (x*y=w493:dbl)
              n282 = Multiply(x=w493, y=w492) -> (x*y=w491:dbl)
              n283 = Sine(x=w491) -> (sin(x)=w490:dbl)
              n284 = Multiply(x=w490, y="Osc. amp. (V)") -> (x*y=w488:dbl)
